vi "MMEM_STOR_CIT_FORM_C.vi"(0 "VISA IN":refnum<visa-resource-name>, 5 "error in":errorcluster, 7 "Traces":string(combo)="AUTO") -> (14 "VISA Out":refnum<visa-resource-name>, 19 "error out":errorcluster)   [LabVIEW 2018, in "PNA-X.lvlib"]
doc: "MMEMory:STORe:CIT:FORMat statements. Choose from: \nMA - Linear Magnitude / degrees \nDB - Log Magnitude / degrees \nRI - Real / Imaginary \nAUTO - Format in which the trace is already displayed. If other than Log \nMag, Linear Magnitude, or Real/Imag, then the format will be in Real/Imag. \nExamples MMEM:STOR:TRAC:FORM:CIT MA \nQuery Syntax MMEMory:STORe:TRACe:FORMat:CITifile? \nReturn Type Character \nDefault Auto'"
uses:
  PNA-X.lvlib
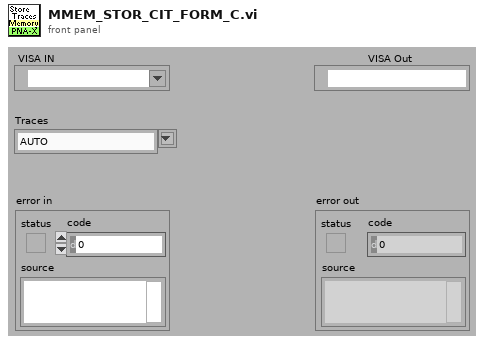
[diagram p1: front panel]
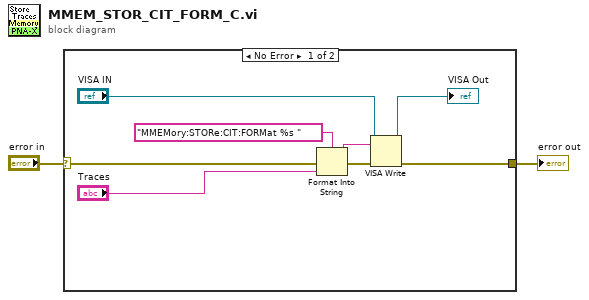
[diagram p0: block diagram]
diagram:
  n1 = case shown="No Error" "error in" {
    selector: "error in" -> [w10 w11]
    tunnel: [w5 w11] -> w1
    frame No Error {
      n2 = Format Into String(format string="MMEMory:STORe:CIT:FORMat %s " ("Cmdline"), error in=w10, "Traces") -> (resulting string=w8:string, error out=w9:errorcluster)  [unwired: 1 in]
      n3 = VISA Write(VISA resource name="VISA IN", write buffer=w8, error in (no error)=w9) -> (VISA resource name out=→"VISA Out":refnum<visa-resource-name>, error out=w5:errorcluster)  [unwired: 1 out]
    }
    frame Error {
    }
  }
  "error out" <- w1
